vi "Random_signal_activity9.vi"() -> ()   [LabVIEW 2025]
panel:
  in  "Loop delay":dbl(knob) scale=0.0..2.0
  out "RandomSignal":dbl(graph)
  in  "Enable":bool
  # "off"
  # "on"
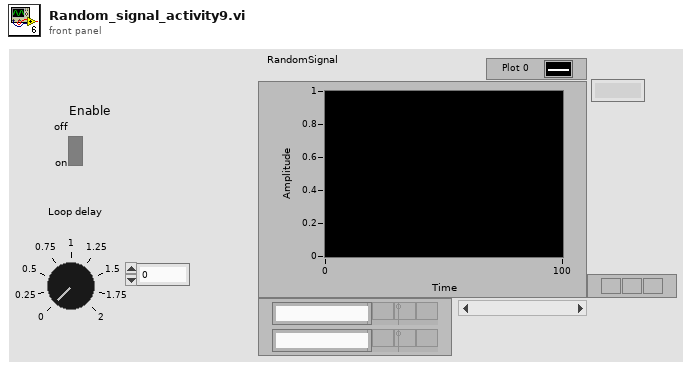
[diagram p1: front panel]
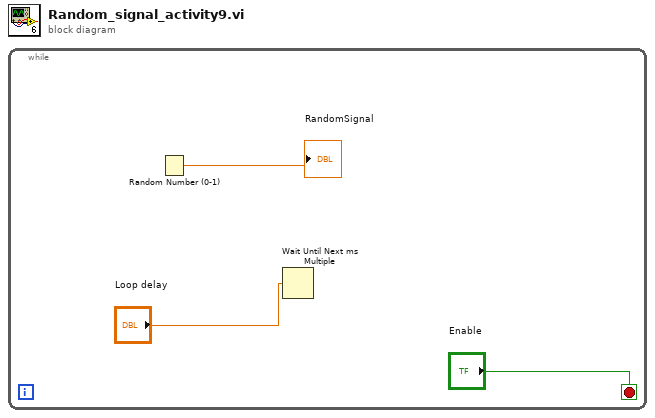
[diagram p0: block diagram]
diagram:
  n1 = while {
    stop <- "Enable" stop-if-true
    n2 = Random Number (0-1)() -> (number: 0 to 1=→"RandomSignal":dbl)
    n3 = Wait Until Next ms Multiple(millisecond multiple="Loop delay") -> ()  [unwired: 1 out]
  }
